vi "forceOutputState.vi"(8 "error in (no error)":errorcluster, 9 "calibratedValues":dbl[](array[numeric]), 10 "channel_addresses":string[](array[string]), 11 "HamegHMPSupply in":refnum<class "HamegHMPSupply.lvclass">) -> (0 "error out":errorcluster, 3 "HamegHMPSupply out":refnum<class "HamegHMPSupply.lvclass">)   [LabVIEW 2011, in "Hardware.lvlib" / "Channels.lvlib" / "HamegHMPSupply.lvclass"]
uses:
  HamegHMPSupply.lvclass
  HamegHMPSupply.lvclass/HamegHMPSupply.ctl
  AnalogOutput.lvclass
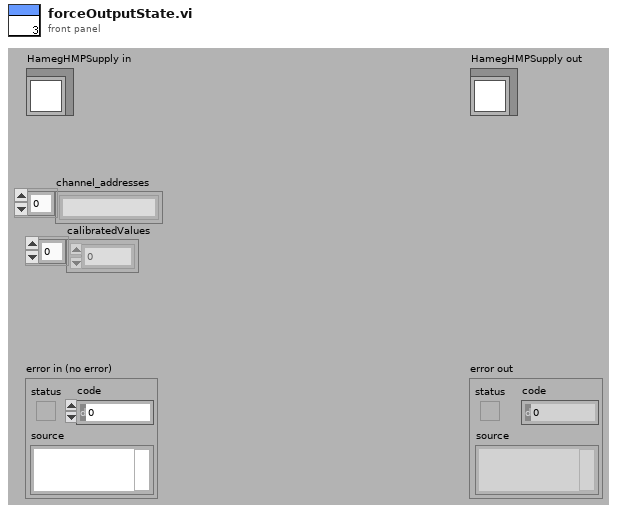
[diagram p1: front panel]
types:
  T1 = cluster{"VoltageLimit":dbl, "CurrentLimit":dbl}[]
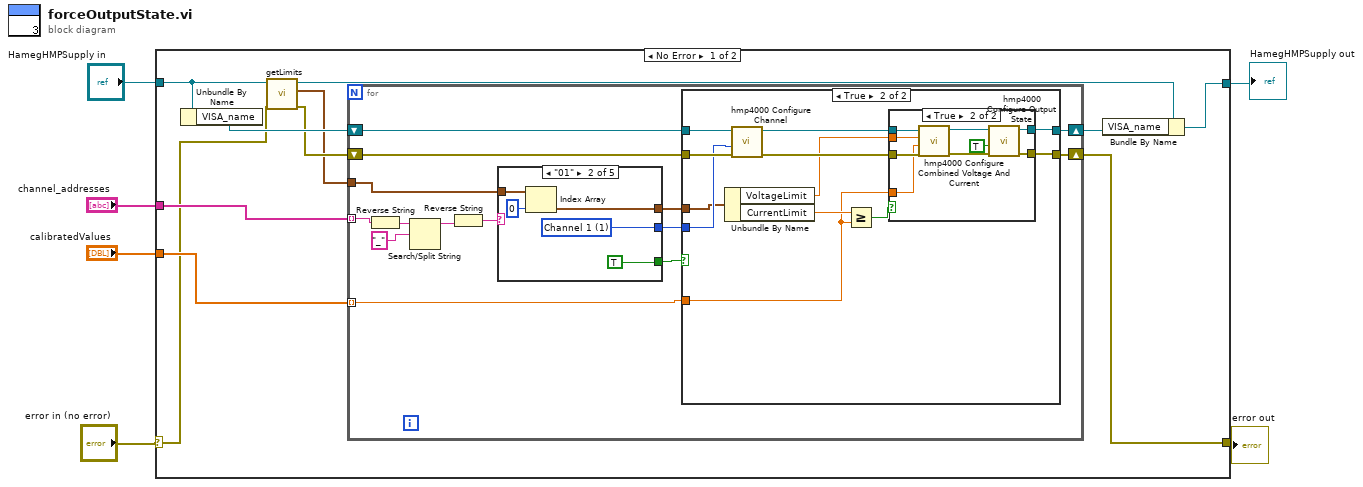
[diagram p0: block diagram]
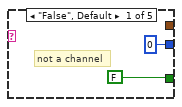
[diagram p4: hidden frame]
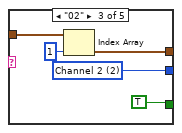
[diagram p5: hidden frame]
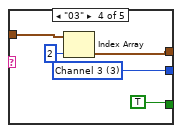
[diagram p6: hidden frame]
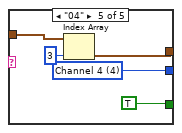
[diagram p7: hidden frame]
diagram:
  n1 = case shown="No Error" "error in (no error)" {
    selector: "error in (no error)" -> [w12 w79]
    tunnel: [w15 w79] -> w5
    tunnel: [w7 w80] -> w1
    tunnel: "HamegHMPSupply in" -> [w13 w80]
    tunnel: "channel_addresses" -> [w16 _]
    tunnel: "calibratedValues" -> [w14 _]
    frame No Error {
      n2 = Unbundle By Name(w13) -> ("VISA_name"=w17:refnum<visa-resource-name>)
      n3 = call "getLimits.vi"("error in (no error)"=w12, "AnalogOutput in"=w13) -> ("error out"=w11:errorcluster, "Limits"=w10:T1, "AnalogOutput out"=w9:refnum<class "HamegHMPSupply.lvclass">)  [unwired: 7 in]
      n4 = for {
        shift-right: [w27] -> w8
        shift-left: w17 -> [w31]
        shift-right: [w26] -> w15
        shift-left: w11 -> [w30]
        tunnel: w16 -> [w23] mode=indexing
        tunnel: w14 -> [w25] mode=indexing
        tunnel: w10 -> [w19]
        n5 = Reverse String(1:w23) -> (0:w22:string)
        n6 = Search/Split String(string=w22, search string/char (-)="_") -> (substring before match=w20:string)  [unwired: 1 in, 2 out]
        n7 = Reverse String(1:w20) -> (0:w21:string)
        n8 = case shown="\"01\"" w21 {
          tunnel: [0 ("Channel (Channel 1)") w63 w68 w73 w78] -> w28
          tunnel: [FALSE TRUE TRUE TRUE TRUE] -> w29
          tunnel: w19 -> [_ w61 w65 w70 w75]
          tunnel: [_ w59 w64 w69 w74] -> w18
          frame "False", Default {
            # "not a channel"
          }
          frame "01" {
            w63 = 1 items=["Channel 1"=1, "Channel 2"=2, "Channel 3"=3, "Channel 4"=4] ("Channel (Channel 1)")
            n9 = Index Array(array=w61, index=0) -> (element=w59:cluster{"VoltageLimit":dbl, "CurrentLimit":dbl})
          }
          frame "02" {
            w68 = 2 items=["Channel 1"=1, "Channel 2"=2, "Channel 3"=3, "Channel 4"=4] ("Channel (Channel 1)")
            n10 = Index Array(array=w65, index=1) -> (element=w64:cluster{"VoltageLimit":dbl, "CurrentLimit":dbl})
          }
          frame "03" {
            w73 = 3 items=["Channel 1"=1, "Channel 2"=2, "Channel 3"=3, "Channel 4"=4] ("Channel (Channel 1)")
            n11 = Index Array(array=w70, index=2) -> (element=w69:cluster{"VoltageLimit":dbl, "CurrentLimit":dbl})
          }
          frame "04" {
            w78 = 4 items=["Channel 1"=1, "Channel 2"=2, "Channel 3"=3, "Channel 4"=4] ("Channel (Channel 1)")
            n12 = Index Array(array=w75, index=3) -> (element=w74:cluster{"VoltageLimit":dbl, "CurrentLimit":dbl})
          }
        }
        n13 = case shown="True" w29 {
          tunnel: w31 -> [w33 w45]
          tunnel: w30 -> [w32 w44]
          tunnel: w28 -> [_ w43]
          tunnel: [w33 w42] -> w27
          tunnel: [w32 w41] -> w26
          tunnel: w25 -> [_ w34]
          tunnel: w18 -> [_ w38]
          frame False {
          }
          frame True {
            n14 = Unbundle By Name(w38) -> ("VoltageLimit"=w35:dbl, "CurrentLimit"=w36:dbl)
            n15 = call <instrlib>:"hmp4000 Configure Channel.vi"("error in (no error)"=w44, "Channel (Channel 1)"=w43, "VISA resource name"=w45) -> ("error out"=w40:errorcluster, "VISA resource name out"=w39:refnum<visa-resource-name>)  [unwired: 7 in]
            n16 = Greater Or Equal?(x=w36, y=w34) -> (x >= y?=w37:bool)
            n17 = case shown="True" w37 {
              tunnel: [w47 w55] -> w42
              tunnel: [w46 w54] -> w41
              tunnel: w40 -> [w46 w51]
              tunnel: w39 -> [w47 w50]
              tunnel: w35 -> [_ w49]
              tunnel: w34 -> [_ w48]
              frame False {
              }
              frame True {
                n18 = call <instrlib>:"hmp4000 Configure Combined Voltage And Current.vi"("error in (no error)"=w51, "Current (0.0)"=w48, "Voltage (0.0)"=w49, "VISA resource name"=w50) -> ("error out"=w52:errorcluster, "VISA resource name out"=w53:refnum<visa-resource-name>)  [unwired: 6 in]
                n19 = call <instrlib>:"hmp4000 Configure Output State.vi"("error in (no error)"=w52, "Output State (Off)"=TRUE, "VISA resource name"=w53) -> ("error out"=w54:errorcluster, "VISA resource name out"=w55:refnum<visa-resource-name>)  [unwired: 7 in]
              }
            }
          }
        }
      }
      n20 = Bundle By Name(cluster=w9, "VISA_name"=w8) -> (w7:refnum<class "HamegHMPSupply.lvclass">)
    }
    frame Error {
    }
  }
  "error out" <- w5
  "HamegHMPSupply out" <- w1
